vi "Parse Systems.vi"(8 "error in (no error)":errorcluster, 9 "server url in":string, 10 "Asset stats in":T2, 11 "Refnum in":T1) -> (0 "error out":errorcluster, 2 "Asset stats out":T2, 3 "Refnum out":T1)   [LabVIEW 2020]
uses:
  <vilib>/httpClient/ClientHandle.ctl
  <vilib>/httpClient/LabVIEWHTTPClient.lvlib
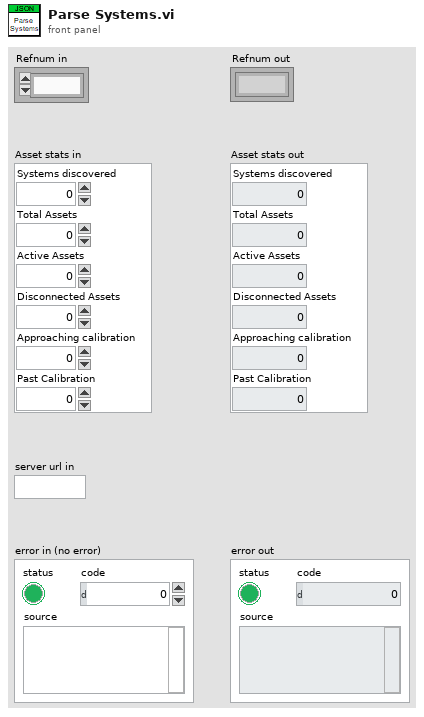
[diagram p1: front panel]
types:
  T1 = typedef "LabVIEWHTTPClient.lvlib/ClientHandle.ctl" = refnum<k1>
  T2 = cluster{"Systems discovered":i32, "Total Assets":i32, "Active Assets":i32, "Disconnected Assets":i32, "Approaching calibration ":i32, "Past Calibration":i32}
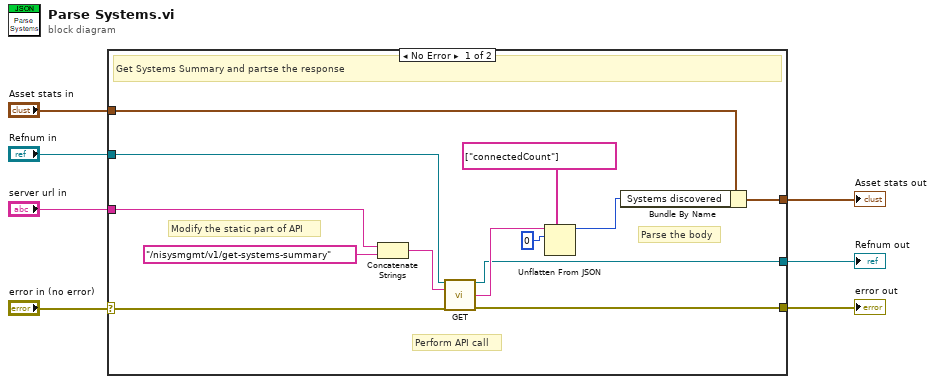
[diagram p0: block diagram]
diagram:
  n1 = case shown="No Error" "error in (no error)" {
    selector: "error in (no error)" -> [w9 w23]
    tunnel: [w19 w21] -> w7
    tunnel: "server url in" -> [w18 _]
    tunnel: "Refnum in" -> [w17 w22]
    tunnel: [w11 w22] -> w4
    tunnel: [w10 w23] -> w3
    tunnel: "Asset stats in" -> [w8 w21]
    frame No Error {
      # "Parse the body"
      # "Perform API call"
      # "Modify the static part of API"
      # "Get Systems Summary and partse the response"
      n2 = Concatenate Strings(w18, "/nisysmgmt/v1/get-systems-summary" ("Get System count API")) -> (w16:string)
      n3 = call <vilib>:"GET.vi"("client handle"=w17, "url"=w16, "error in (no error)"=w9) -> ("client handle out"=w11:T1, "body"=w12:string, "error out"=w10:errorcluster)  [unwired: 9 in, 1 out]
      n4 = Unflatten From JSON(path=string[] ["connectedCount"], JSON string=w12, type and defaults=0) -> (value=w20:i32)  [unwired: 4 in, 1 out]
      n5 = Bundle By Name(cluster=w8, "Systems discovered"=w20) -> (w19:T2)
    }
    frame Error {
    }
  }
  "Asset stats out" <- w7
  "Refnum out" <- w4
  "error out" <- w3
